vi "IndoorMonitoring_Main.vi"() -> ()   [LabVIEW 2014]
uses:
  IndoorData_class/DebugData.ctl
  IndoorData_class/ActualValues.ctl
  NodeConfiguration_class/Config.ctl
  <vilib>/Platform/TimedLoop/XDataNode/timing_clust.ctl
  <vilib>/Platform/TimedLoop/XDataNode/nitl_modes.ctl
  <vilib>/Platform/TimedLoop/XDataNode/wakeup.ctl
  <vilib>/MakerHub/LINX/Public/Peripherals/Digital/Digital Write 1 Chan.vi
  <vilib>/MakerHub/LINX/Public/Peripherals/Digital/Digital Write N Chans.vi
  <vilib>/MakerHub/LINX/Private/Local IO/LinxDigitalWrite.vi
  <vilib>/MakerHub/LINX/Public/Utilities/Check Channel.vi
  <vilib>/MakerHub/LINX/Private/Local IO/Handle Errors.vi
  <vilib>/MakerHub/LINX/Public/Utilities/Open Local.vi
  <vilib>/MakerHub/LINX/Private/Utilties/Generate Error.vi
  <vilib>/platform/TimedLoop/XDataNode/XDataNode.xnode
  NodeConfiguration_class/NodeConfiguration.lvclass
  Sensor_SHT21/SHT21_class/SHT21.lvclass
  IndoorData_class/IndoorData.lvclass
  <vilib>/Platform/TimedLoop/XDataNode/XDNodeRunTimeDep.lvlib
  <vilib>/MakerHub/LINX/LMH-LINX.lvlib
panel:
  out "Config":T1
  out "ActualValues":T2
  out "DebugData":T3
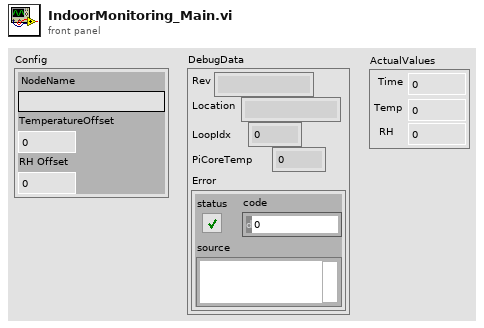
[diagram p1: front panel]
types:
  T1 = typedef "NodeConfiguration.lvclass/Config.ctl" = cluster{"NodeName":string, "TemperatureOffset":dbl, "RH Offset":dbl}
  T2 = typedef "IndoorData.lvclass/ActualValues.ctl" = cluster{"Time":dbl, "Temp":dbl, "RH":dbl}
  T3 = typedef "IndoorData.lvclass/DebugData.ctl" = cluster{"Rev":string, "Location":string, "LoopIdx":i32, "PiCoreTemp":dbl, "Error":errorcluster}
  T4 = typedef "LMH-LINX.lvlib/LINX Ref.ctl" = cluster{"IO":T5, "Interface":T6, "LINX Device Config":T7}
  T5 = typedef "LMH-LINX.lvlib/Platform.ctl" = enum16{"Remote", "Local"}
  T6 = typedef "LMH-LINX.lvlib/Interface.ctl" = enum16{"Serial", "TCP"}
  T7 = typedef "LMH-LINX.lvlib/Device.lvlib/LINX Device Config.ctl" = cluster{"Interface":T6, "COM Port":refnum<visa-resource-name>, "TCP Configuration":T8, "Device Family":u8, "Device ID":u8, "Device Name":string, "TCP Ref":refnum<k5>, "Channels":T9}
  T8 = typedef "LMH-LINX.lvlib/Device.lvlib/TCP Config.ctl" = cluster{"IP Address":string, "Port":u16}
  T9 = typedef "LMH-LINX.lvlib/Channels.ctl" = cluster{"DI":u8[], "DO":u8[], "AI":u8[], "AO":u8[], "PWM":u8[], "QE":u8[], "UART":u8[], "I2C 2":u8[], "SPI":u8[], "CAN":u8[], "Servo":u8[], "AI Ref (V)":dbl, "AI Resolution (Bits)":u8, "AO Ref (V)":dbl, "AO Resolution (Bits)":u8}
  T10 = typedef "XDNodeRunTimeDep.lvlib/timing_clust.ctl" = cluster{"Expected End [f-1]":u64, "Actual End [f-1]":u64, "Finished Late? [f-1]":bool, "Expected End [i-1]":u64, "Actual End [i-1]":u64, "Finished Late? [i-1]":bool, "Expected Start [i]":u64, "Actual Start [i]":u64, "Expected Start [f]":u64, "Actual Start [f]":u64, "Source Name":string, "Structure Name":string, "Period":i64, "Deadline":i64, "Offset":i64, "Start":i64, "Priority":i32, "Timeout":i32, "Mode":T11, "Wakeup Reason":T12, "Error":errorcluster, "Source Type":string, "Secondary Source Type":string, "Global End Time":u64, "Global Start Time":u64, "Frame Duration":u64, "Iteration Duration":u64, "Assigned CPU":i32, "I/O Scan Engine Mode":u32}
  T11 = typedef "XDNodeRunTimeDep.lvlib/nitl_modes.ctl" = enum32{"No Change", "Process missed periods, maintain original phase", "Discard missed periods, maintain original phase", "Process missed periods, ignore original phase", "Discard missed periods, ignore original phase"}
  T12 = typedef "XDNodeRunTimeDep.lvlib/wakeup.ctl" = enum32{"Normal", "Aborted", "Asynchronous wakeup", "Timing source error", "Timed loop error", "Timeout"}
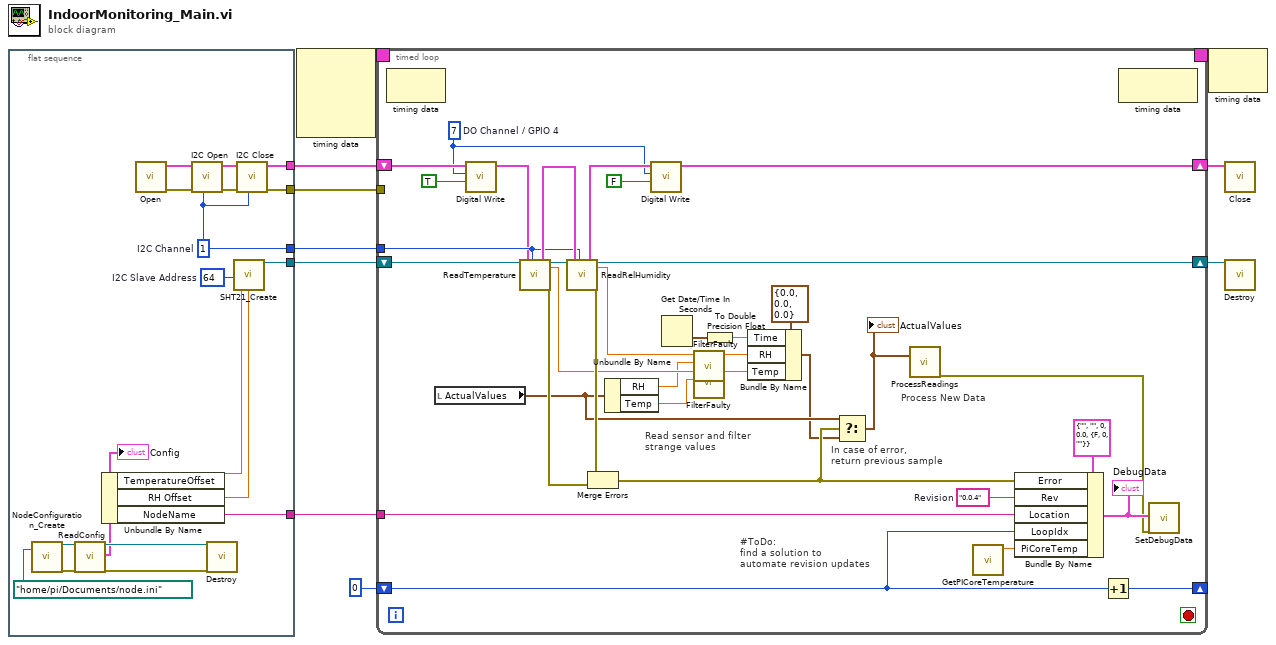
[diagram p0: block diagram]
diagram:
  n1 = flat-sequence {
    tunnel: [w24] -> w7
    tunnel: [w23] -> w6
    tunnel: [w22] -> w4
    tunnel: [w20] -> w2
    tunnel: [w15] -> w1
    frame #0 {
      w21 = u8 64  # I2C Slave Address
      w20 = u8 1  # I2C Channel
      n2 = call "NodeConfiguration_Create.vi"("ConfigFile"=path "/home/pi/Documents/node.ini") -> ("reference out"=w17:refnum<class "NodeConfiguration.lvclass">, "error out"=w16:errorcluster)  [unwired: 17 in]
      n3 = call-dynamic "ReadConfig.vi"("reference in"=w17, "error in (no error)"=w16) -> ("reference out"=w19:refnum<class "NodeConfiguration.lvclass">, "Config"=w11:T1, "error out"=w18:errorcluster)  [unwired: 15 in]
      "Config" <- w11
      n4 = Unbundle By Name(w11) -> ("TemperatureOffset"=w13:dbl, "RH Offset"=w12:dbl, "NodeName"=w15:string)
      n5 = call-poly <vilib>:"Open.vi"() -> ("Error Out"=w26:errorcluster, "LINX Resource"=w28:T4)  [unwired: 9 in, 1 out]
      n6 = call <vilib>:"I2C Open.vi"("I2C Channel (0)"=w20, "Error In"=w26, "LINX Resource"=w28) -> ("Error Out"=w25:errorcluster, "LINX Resource"=w27:T4)  [unwired: 7 in]
      n7 = call-dynamic "Destroy.vi"("reference in"=w19, "error in (no error)"=w18) -> ()  [unwired: 16 in, 2 out]
      n8 = call "SHT21_Create.vi"("I2C Slave Address (0)"=w21, "T Offset"=w13, "RH Offset"=w12) -> ("reference out"=w22:refnum<class "SHT21.lvclass">)  [unwired: 15 in, 1 out]
      n9 = call <vilib>:"I2C Close.vi"("I2C Channel (0)"=w20, "Error In"=w25, "LINX Resource"=w27) -> ("Error Out"=w23:errorcluster, "LINX Resource"=w24:T4)  [unwired: 7 in]
    }
  }
  n10 = node-c288() -> (w10:T10)  [unwired: 4 in]
  n11 = timed-loop {
    timing: w10 -> [_]
    timing-out: [_] -> w9
    shift-right: [w60] -> _
    shift-left: 0 -> [w40]
    shift-right: [w44] -> w5
    shift-left: w7 -> [w48]
    tunnel: w6 -> [_]
    shift-right: [w56] -> w3
    shift-left: w4 -> [w58]
    tunnel: w2 -> [w54]
    tunnel: w1 -> [w42]
    stop <- _ stop-if-true
    w29 = u8 7  # DO Channel / GPIO 4
    w59 = "0.0.4"  # Revision
    # "#ToDo:\nfind a solution to\nautomate revision updates"
    # "Process New Data"
    # "Read sensor and filter\nstrange values"
    # "In case of error,\nreturn previous sample"
    n12 = node-c288() -> ()  [unwired: 1 in, 1 out]
    n13 = local read "ActualValues"() -> (w32:T2)
    n14 = call-poly <vilib>:"Digital Write.vi"("Output Value"=TRUE, "DO Channel"=w29, "LINX Resource"=w48) -> ("LINX Resource"=w47:T4)  [unwired: 7 in, 1 out]
    n15 = call-dynamic "ReadTemperature.vi"("reference in"=w58, "LINX Resource"=w47, "I2C Channel (0)"=w54) -> ("LINX Resource"=w55:T4, "reference out"=w57:refnum<class "SHT21.lvclass">, "Temperature"=w36:dbl, "error out"=w53:errorcluster)  [unwired: 12 in, 1 out]
    n16 = call-dynamic "ReadRelHumidity.vi"("reference in"=w57, "LINX Resource"=w55, "I2C Channel (0)"=w54) -> ("LINX Resource"=w45:T4, "reference out"=w56:refnum<class "SHT21.lvclass">, "RH"=w39:dbl, "error out"=w52:errorcluster)  [unwired: 12 in, 1 out]
    n17 = Merge Errors(w52, w53) -> (w33:errorcluster)
    n18 = Unbundle By Name(w32) -> ("RH"=w35:dbl, "Temp"=w34:dbl)
    n19 = call-poly <vilib>:"Digital Write.vi"("Output Value"=FALSE, "DO Channel"=w29, "LINX Resource"=w45) -> ("LINX Resource"=w44:T4)  [unwired: 7 in, 1 out]
    n20 = Get Date/Time In Seconds() -> (seconds since 1Jan1904=w49:timestamp)
    n21 = call "FilterFaulty.vi"("Prev. Measurement In"=w35, "Measurement In"=w39) -> ("Measurement Out"=w38:dbl)  [unwired: 9 in]
    n22 = call "FilterFaulty.vi"("Prev. Measurement In"=w34, "Measurement In"=w36) -> ("Measurement Out"=w37:dbl)  [unwired: 9 in]
    n23 = To Double Precision Float(number=w49) -> (double precision float=w50:dbl)
    n24 = Bundle By Name(cluster=T2 {"Time"=0.0, "Temp"=0.0, "RH"=0.0} ("ActualValues"), "Time"=w50, "RH"=w38, "Temp"=w37) -> (w31:T2)
    n25 = Select(t=w32, s=w33, f=w31) -> (s? t:f=w30:T2)
    "ActualValues" <- w30
    n26 = call "ProcessReadings.vi"("ActualValues"=w30) -> ("error out"=w41:errorcluster)  [unwired: 18 in]
    n27 = call "GetPICoreTemperature.vi"() -> ("PICoreTemp"=w63:dbl)  [unwired: 10 in, 1 out]
    n28 = Bundle By Name(cluster=T3 {"Rev"="", "Location"="", "LoopIdx"=0, "PiCoreTemp"=0.0, "Error"={"status"=FALSE, "code"=0, "source"=""}} ("DebugData"), "Error"=w33, "Rev"=w59, "Location"=w42, "LoopIdx"=w40, "PiCoreTemp"=w63) -> (w62:T3)
    "DebugData" <- w62
    n29 = Increment(x=w40) -> (x+1=w60:i32)
    n30 = node-c288() -> ()  [unwired: 1 in, 1 out]
    n31 = call "SetDebugData.vi"("DebugData"=w62, "error in (no error)"=w41) -> ()  [unwired: 17 in, 1 out]
  }
  n32 = node-c288(w9) -> ()  [unwired: 1 out]
  n33 = call <vilib>:"Close.vi"("LINX Resource"=w5) -> ()  [unwired: 10 in, 1 out]
  n34 = call-dynamic "Destroy.vi"("reference in"=w3) -> ()  [unwired: 17 in, 2 out]
